vi "pochodna.vi"(10 "współczynniki":dbl[](array[numeric]), 11 "rząd":i32) -> (3 "pochodna":dbl[](array[numeric]))   [LabVIEW 2020]
doc: "Obliczanie pochodnej"
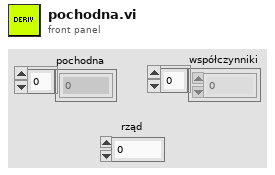
[diagram p1: front panel]
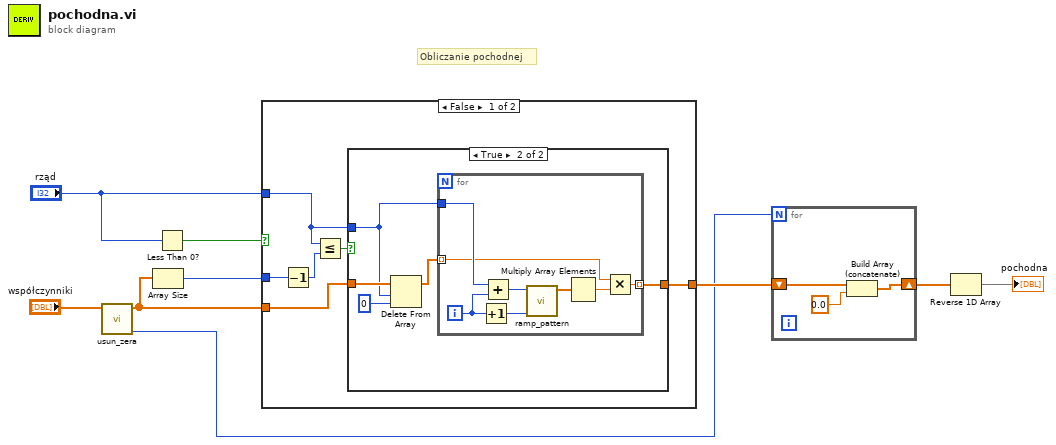
[diagram p0: block diagram]
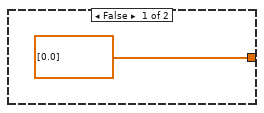
[diagram p2: hidden frame]
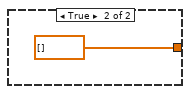
[diagram p3: hidden frame]
diagram:
  # "Obliczanie pochodnej"
  n1 = call "usun_zera.vi"("Tablica współczynników"="współczynniki") -> ("ilość zer"=w3:i32, "Współczynniki"=w9:dbl[])  [unwired: 9 in]
  n2 = Array Size(array=w9) -> (size(s)=w6:i32)
  n3 = Less Than 0?(x="rząd") -> (x < 0?=w7:bool)
  n4 = case shown="False" w7 {
    tunnel: w9 -> [w15 _]
    tunnel: w6 -> [w12 _]
    tunnel: "rząd" -> [w11 _]
    tunnel: [w10 dbl[] []] -> w5
    frame False {
      n5 = Decrement(x=w12) -> (x-1=w13:i32)
      n6 = Less Or Equal?(x=w11, y=w13) -> (x <= y?=w14:bool)
      n7 = case shown="True" w14 {
        tunnel: w15 -> [_ w21]
        tunnel: w11 -> [_ w19]
        tunnel: [dbl[] [0.0] ("Polynomial dp(s)/ds") w17] -> w10
        frame False {
        }
        frame True {
          n8 = Delete From Array(array=w21, length=w19, index=0) -> (array with subset deleted=w18:dbl[])  [unwired: 1 out]
          n9 = for {
            tunnel: w18 -> [w27] mode=indexing
            tunnel: w19 -> [w28]
            tunnel: [w25] -> w17 mode=indexing
            i -> [w29]
            n10 = Increment(x=w29) -> (x+1=w22:i32)
            n11 = Add(x=w28, y=w29) -> (x+y=w24:i32)
            n12 = call "ramp_pattern.vi"("start"=w22, "end"=w24) -> ("schodki"=w23:dbl[])  [unwired: 9 in]
            n13 = Multiply Array Elements(1:w23) -> (0:w26:dbl)
            n14 = Multiply(x=w27, y=w26) -> (x*y=w25:dbl)
          }
        }
      }
    }
    frame True {
    }
  }
  n15 = for {
    N: w3 -> [_]
    shift-right: [w32] -> w2
    shift-left: w5 -> [w33]
    n16 = Build Array (concatenate)(w33, 0.0) -> (w32:dbl[])
  }
  n17 = Reverse 1D Array(array=w2) -> (reversed array=→"pochodna":dbl[])
